vi "Log_chart_images.vi"(9 "image data":T1, 11 "JSON DEV":string) -> (3 "2D Picture":picture)   [LabVIEW 2015]
uses:
  <vilib>/picture/picture.llb/imagedata.ctl
  Share Data/uPower_kit.ctl
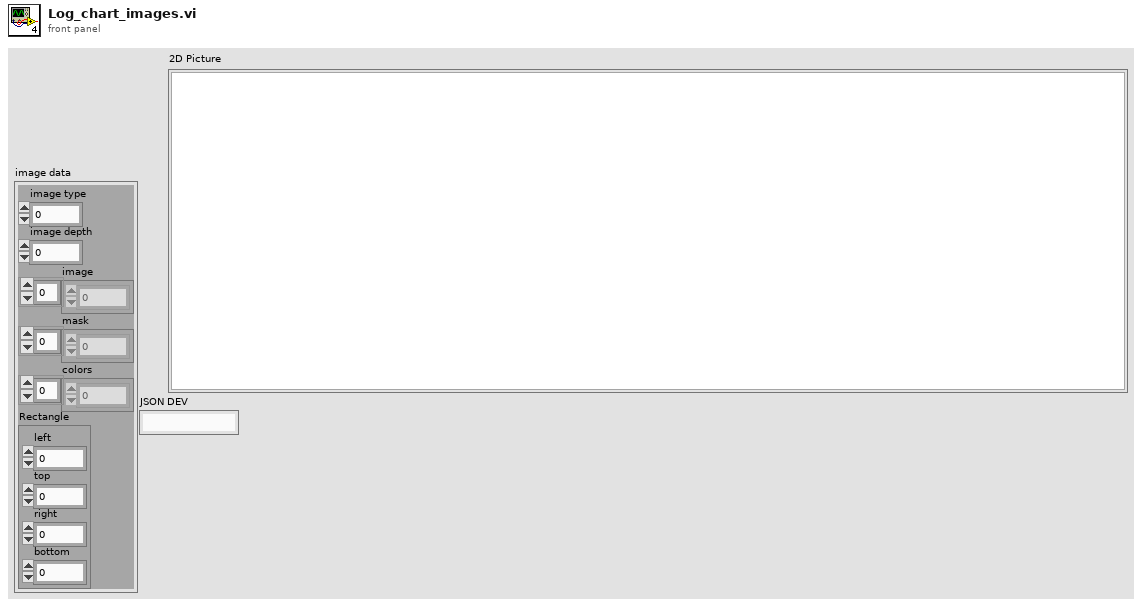
[diagram p1: front panel]
types:
  T1 = typedef "imagedata.ctl" = cluster{"image type":i32, "image depth":i32, "image":u8[], "mask":u8[], "colors":u32[], "Rectangle":cluster{"left":i16, "top":i16, "right":i16, "bottom":i16}}
  T2 = typedef "uPower_kit.ctl" = cluster{"DEV":string, "BUSY":bool, "VBAT":dbl, "OUTPUT":bool, "LAST_RESULT":dbl, "DURATION":u16, "TRIGGER":bool, "RANGE":string, "Vsource":dbl, "FW":string, "Mode":string}
  T3 = enum16{"User-specified Font", "Application Font", "System Font", "Dialog Font"}
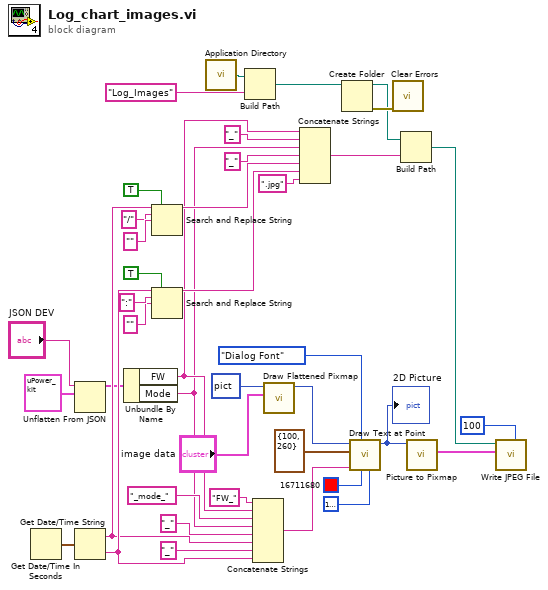
[diagram p0: block diagram]
diagram:
  n1 = Get Date/Time In Seconds() -> (seconds since 1Jan1904=w24:timestamp)
  n2 = Unflatten From JSON(JSON string="JSON DEV", type and defaults=T2 {"DEV"="", "BUSY"=FALSE, "VBAT"=0.0, "OUTPUT"=FALSE, "LAST_RESULT"=0.0, "DURATION"=0, "TRIGGER"=FALSE, "RANGE"="", "Vsource"=0.0, "FW"="", "Mode"=""} ("DEV_BUSY")) -> (value=w3:T2)  [unwired: 5 in, 1 out]
  n3 = Get Date/Time String(seconds (now)=w24) -> (date string=w29:string, time string=w36:string)  [unwired: 2 in]
  n4 = Unbundle By Name(w3) -> ("FW"=w2:string, "Mode"=w1:string)
  n5 = Search and Replace String(replace all?=TRUE ("replace all? (F)"), input string=w29, search string="/", replace string="" ("replace string (\"\")")) -> (result string=w38:string)  [unwired: 4 in, 3 out]
  n6 = Search and Replace String(replace all?=TRUE ("replace all? (F)"), input string=w36, search string=":", replace string="" ("replace string (\"\")")) -> (result string=w37:string)  [unwired: 4 in, 3 out]
  n7 = call <vilib>:"Application Directory.vi"() -> ("Application Directory"=w14:path)
  n8 = Build Path(base path=w14, name or relative path="Log_Images") -> (appended path=w16:path)
  n9 = Concatenate Strings("FW_" ("string"), w2, "_mode_" ("string"), w1, "_" ("string"), w29, "_" ("string"), w36) -> (w23:string)
  n10 = call <vilib>:"Draw Flattened Pixmap.vi"("image data"="image data", "picture"=picture data[5B]) -> ("new picture"=w7:picture)  [unwired: 7 in]
  n11 = Concatenate Strings(w2, "_" ("string"), w1, "_" ("string"), w38, w37, ".jpg" ("string")) -> (w28:string)
  n12 = Create Folder(path (use dialog)=w16) -> (created path=w17:path, error out=w19:errorcluster)  [unwired: 2 in, 1 out]
  n13 = call <vilib>:"Draw Text at Point.vi"("BG color(transparent)"=u32 16777216, "text color(black)"=u32 16711680, "desired font(Application)"=T3."Dialog Font", "text"=w23, "origin"=cluster{"x":i16, "y":i16} {"x"=100, "y"=260}, "picture"=w7) -> ("new picture"=w12:picture)  [unwired: 4 in, 1 out]
  "2D Picture" <- w12
  n14 = call <vilib>:"Clear Errors.vi"("error in (no error)"=w19) -> ()  [unwired: 5 in, 2 out]
  n15 = Build Path(base path=w17, name or relative path=w28) -> (appended path=w18:path)
  n16 = call <vilib>:"Picture to Pixmap.vi"("picture"=w12) -> ("image data"=w13:T1)  [unwired: 9 in, 1 out]
  n17 = call <vilib>:"Write JPEG File.vi"("quality (80)"=100, "image data"=w13, "path to JPEG file"=w18) -> ()  [unwired: 7 in, 2 out]
